vi "Generate Random Error.vi"(7 "Prob":dbl=0.1, 11 "error in (no error)":errorcluster) -> (15 "error out":errorcluster)   [LabVIEW 2015]
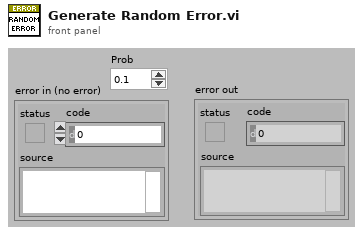
[diagram p1: front panel]
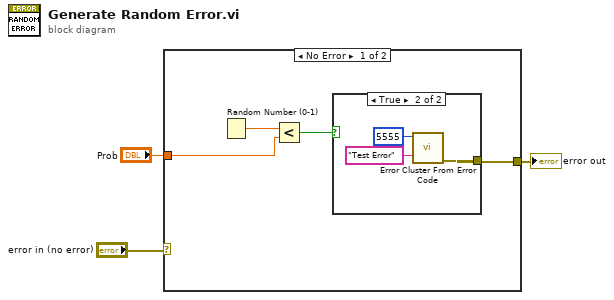
[diagram p0: block diagram]
diagram:
  n1 = case shown="No Error" "error in (no error)" {
    selector: "error in (no error)" -> [_ w11]
    tunnel: [w5 w11] -> w2
    tunnel: "Prob" -> [w4 _]
    frame No Error {
      n2 = Random Number (0-1)() -> (number: 0 to 1=w7:dbl)
      n3 = Less?(x=w7, y=w4) -> (x < y?=w6:bool)
      n4 = case shown="True" w6 {
        tunnel: [_ w8] -> w5
        frame False {
        }
        frame True {
          n5 = call <vilib>:"Error Cluster From Error Code.vi"("error message (\"\")"="Test Error" ("error message (\"\")"), "error code (0)"=5555) -> ("error out"=w8:errorcluster)  [unwired: 7 in]
        }
      }
    }
    frame Error {
    }
  }
  "error out" <- w2
